vi "FS-Simple Duplex.vi"() -> ()   [LabVIEW 2020]
uses:
  <instrlib>/niUSRP/niUSRP Fetch Rx Data (I16).vi
  <instrlib>/niUSRP/niUSRP Write Tx Data (I16).vi
panel:
  out "data":i16[](array[numeric])
  in  "停止 2":bool
  in  "停止":bool
  in  "gain":dbl format="%#_6f"
  in  "carrier frequency":dbl=100000.0 format="%#_6p"
  in  "IQ rate":dbl=100000.0 format="%#_6p"
  in  "number of samples":i64=1000
  in  "device names":refnum<k15>="192.168.1.51"
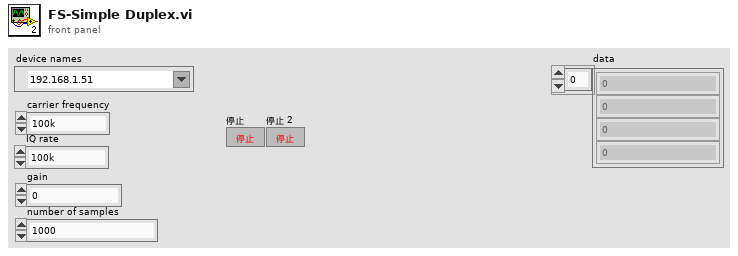
[diagram p1: front panel]
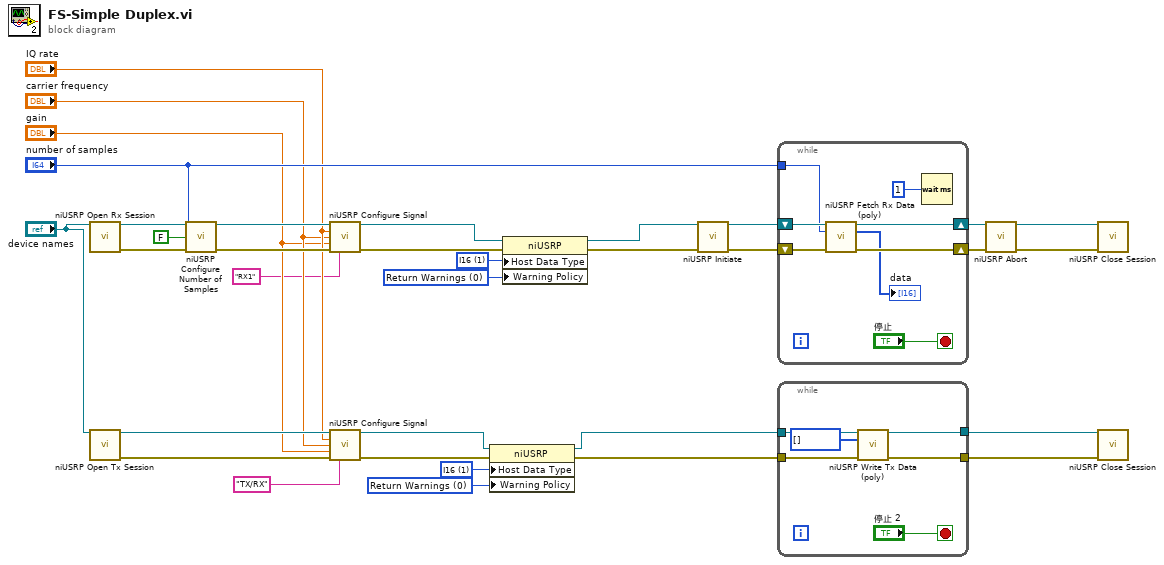
[diagram p0: block diagram]
diagram:
  w1 = 0 items=["Return Warnings", "Return Errors", "Return Success"] ("Configuration:Advanced:Warning Policy")
  w2 = 1 items=["CDB", "I16"] ("Configuration:Advanced:Host Data Type")
  w7 = 0 items=["Return Warnings", "Return Errors", "Return Success"] ("Configuration:Advanced:Warning Policy")
  w8 = 1 items=["CDB", "I16"] ("Configuration:Advanced:Host Data Type")
  n1 = call <instrlib>:"niUSRP Open Rx Session.vi"("device names"="device names") -> ("session handle out"=w34:refnum<k15>, "error out"=w24:errorcluster)  [unwired: 13 in]
  n2 = call <instrlib>:"niUSRP Open Tx Session.vi"("device names"="device names") -> ("session handle out"=w20:refnum<k15>, "error out"=w19:errorcluster)  [unwired: 13 in]
  n3 = call <instrlib>:"niUSRP Configure Number of Samples.vi"("session handle"=w34, "number of samples is finite"=FALSE, "number of samples"="number of samples", "error in (no error)"=w24) -> ("session handle out"=w33:refnum<k15>, "error out"=w25:errorcluster)  [unwired: 10 in]
  n4 = call <instrlib>:"niUSRP Configure Signal.vi"("session handle"=w33, "IQ rate"="IQ rate", "carrier frequency"="carrier frequency", "gain"="gain", "error in (no error)"=w25, "active antenna"="RX1") -> ("session handle out"=w32:refnum<k15>, "error out"=w10:errorcluster)  [unwired: 5 in, 3 out]
  n5 = call <instrlib>:"niUSRP Configure Signal.vi"("session handle"=w20, "IQ rate"="IQ rate", "carrier frequency"="carrier frequency", "gain"="gain", "error in (no error)"=w19, "active antenna"="TX/RX") -> ("session handle out"=w6:refnum<k15>, "error out"=w4:errorcluster)  [unwired: 5 in, 3 out]
  n6 = property class="niUSRP"(reference=w6, error in=w4, "Host Data Type"=w2, "Warning Policy"=w1) -> (reference out=w5:refnum<k15>, error out=w3:errorcluster)
  n7 = property class="niUSRP"(reference=w32, error in=w10, "Host Data Type"=w8, "Warning Policy"=w7) -> (reference out=w11:refnum<k15>, error out=w9:errorcluster)
  n8 = call <instrlib>:"niUSRP Initiate.vi"("session handle"=w11, "error in (no error)"=w9) -> ("session handle out"=w31:refnum<k15>, "error out"=w26:errorcluster)  [unwired: 12 in]
  n9 = while {
    shift-right: [w41] -> w30
    shift-left: w31 -> [w42]
    shift-right: [w40] -> w27
    shift-left: w26 -> [w39]
    tunnel: "number of samples" -> [w36]
    stop <- "停止" stop-if-true
    n10 = call-poly <instrlib>:"niUSRP Fetch Rx Data (poly).vi"("session handle"=w42, "number of samples"=w36, "error in (no error)"=w39) -> ("session handle out"=w41:refnum<k15>, "data"=→"data":i16[], "error out"=w40:errorcluster)  [unwired: 9 in, 1 out]
    n11 = Wait (ms)(milliseconds to wait=u32 1 ("ミリ秒待機時間")) -> ()  [unwired: 1 out]
  }
  n12 = while {
    tunnel: w5 -> [w48]
    tunnel: w3 -> [w47]
    tunnel: [w45] -> w14
    tunnel: [w44] -> w13
    stop <- "停止 2" stop-if-true
    n13 = call-poly <instrlib>:"niUSRP Write Tx Data (poly).vi"("session handle"=w48, "data"=i16[] [], "error in (no error)"=w47) -> ("session handle out"=w45:refnum<k15>, "error out"=w44:errorcluster)  [unwired: 11 in]
  }
  n14 = call <instrlib>:"niUSRP Abort.vi"("session handle"=w30, "error in (no error)"=w27) -> ("session handle out"=w29:refnum<k15>, "error out"=w28:errorcluster)  [unwired: 12 in]
  n15 = call <instrlib>:"niUSRP Close Session.vi"("session handle"=w29, "error in (no error)"=w28) -> ()  [unwired: 13 in, 1 out]
  n16 = call <instrlib>:"niUSRP Close Session.vi"("session handle"=w14, "error in (no error)"=w13) -> ()  [unwired: 13 in, 1 out]
